vi "Format Output Channel List.vi"() -> (0 "Output Channels":string)   [LabVIEW 2013]
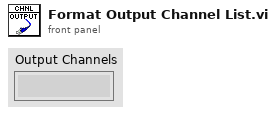
[diagram p1: front panel]
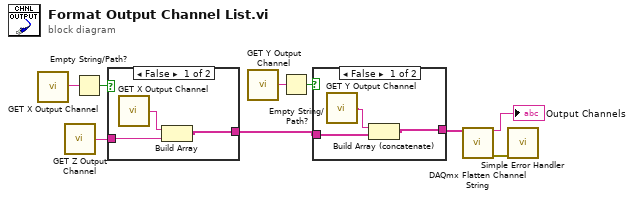
[diagram p0: block diagram]
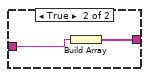
[diagram p3: hidden frame]
diagram:
  n1 = call "GET X Output Channel.vi"() -> ("X Output Channel"=w7:string)
  n2 = call "GET Z Output Channel.vi"() -> ("Z Output Channel"=w1:string)
  n3 = Empty String/Path?(string/path=w7) -> (empty?=w8:bool)
  n4 = case shown="False" w8 {
    tunnel: w1 -> [w12 w13]
    tunnel: [w10 w14] -> w9
    frame False {
      n5 = call "GET X Output Channel.vi"() -> ("X Output Channel"=w11:string)
      n6 = Build Array(w11, w12) -> (w10:string[])
    }
    frame True {
      n7 = Build Array(w13) -> (w14:string[])
    }
  }
  n8 = call "GET Y Output Channel.vi"() -> ("Y Output Channel"=w5:string)
  n9 = Empty String/Path?(string/path=w5) -> (empty?=w6:bool)
  n10 = case shown="False" w6 {
    tunnel: w9 -> [w17 w18]
    tunnel: [w15 w18] -> w4
    frame False {
      n11 = call "GET Y Output Channel.vi"() -> ("Y Output Channel"=w16:string)
      n12 = Build Array (concatenate)(w16, w17) -> (w15:string[])
    }
    frame True {
    }
  }
  n13 = call <vilib>:"DAQmx Flatten Channel String.vi"("names in"=w4) -> ("names out"=→"Output Channels":string, "error out"=w2:errorcluster)  [unwired: 13 in]
  n14 = call <vilib>:"Simple Error Handler.vi"("error in (no error)"=w2) -> ()  [unwired: 4 in, 5 out]
